vi "TestRFGVRoom.vi"() -> (0 "error out":errorcluster, 2 "Pass":bool)   [LabVIEW 2015]
uses:
  LVClasses/Flags/ColorFlags.ctl
  TypeDef/RoomsActionEnum.ctl
  LVClasses/Room/Room.lvclass/Room.ctl
  LVClasses/Room/Read Flags.lvclass.vi
  LVClasses/Flags/Flags.lvclass
  LVClasses/Room/Room.lvclass
panel:
  out "Read Room JSON 2":string
  out "Read Room JSON 1":string
  out "Read Room 2":T1={"Flag State"=[1, 3, 5, 7]}
  out "Read Flag":string
  out "Write Flag":string
  in  "State":bool[](array[boolean])=[FALSE, FALSE, FALSE, FALSE]
  out "Flags Read 1":T1={"Flag State"=[1, 3, 5, 7]}
  out "Flags Write":T1={"Flag State"=[1, 3, 5, 7]}
  out "Flags Read 2":T1={"Flag State"=[1, 3, 5, 7]}
  in  "FGV Room":i32=102
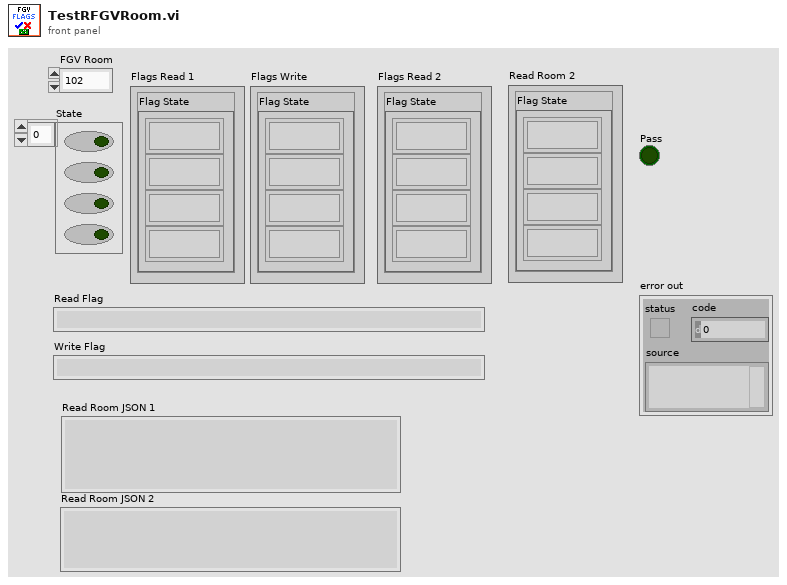
[diagram p1: front panel]
types:
  T1 = typedef "Flags.lvclass/ColorFlags.ctl" = cluster{"Flag State":u8[]}
  T2 = typedef "RoomsActionEnum.ctl" = enum16{"Init", "Add Room", "Remove Room", "Read Room", "Read Flag", "Read Flag State", "Write Flag State", "Read Flag Color", "Write Flag Color", "Read Bed Vacant", "Write Bed Vacant", "Read Personnel", "Add Personnel", "Remove Personnel", "Read Requests", "Add Request", "Remove Request", "Read Beacon ID", "Write Beacon ID", "Write Bed URL", "Read Bed URL", "Read Rooms Numbers", "Write Flag"}
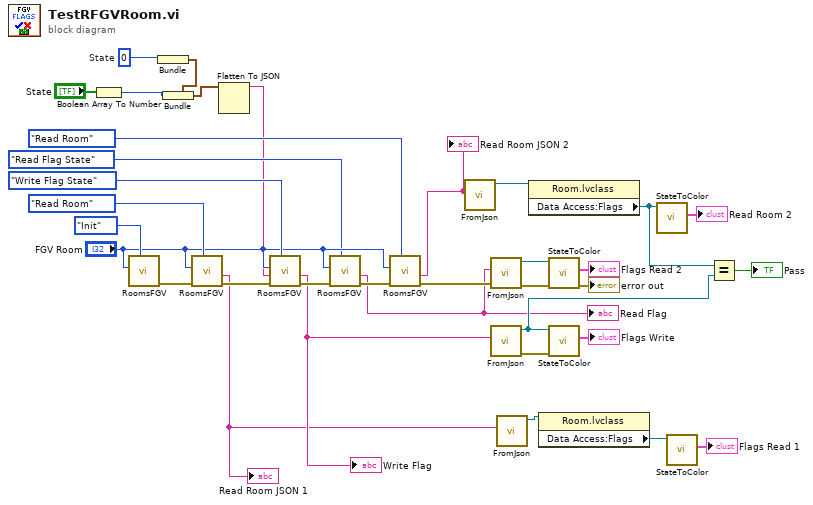
[diagram p0: block diagram]
diagram:
  w5 = u32 0  # State
  n1 = Boolean Array To Number(Boolean array="State") -> (number=w4:u32)
  n2 = call "RoomsFGV.vi"("Actions"=RoomsActionEnum."Init", "Room"="FGV Room") -> ("error out"=w34:errorcluster)  [unwired: 8 in, 1 out]
  n3 = Bundle("State"=w5) -> (w2:cluster{"State":u32})  [unwired: 1 in]
  n4 = Bundle(cluster=w2, "State"=w4) -> (w3:cluster{"State":u32})
  n5 = call "RoomsFGV.vi"("Actions"=RoomsActionEnum."Read Room", "error in (no error)"=w34, "Room"="FGV Room") -> ("error out"=w33:errorcluster, "Data Out"=w12:string)  [unwired: 7 in]
  "Read Room JSON 1" <- w12
  n6 = Flatten To JSON(anything=w3) -> (JSON string=w1:string)  [unwired: 2 in, 1 out]
  n7 = call "RoomsFGV.vi"("Actions"=RoomsActionEnum."Write Flag State", "error in (no error)"=w33, "Data In"=w1, "Room"="FGV Room") -> ("error out"=w32:errorcluster, "Data Out"=w23:string)  [unwired: 6 in]
  "Write Flag" <- w23
  n8 = call "RoomsFGV.vi"("Actions"=RoomsActionEnum."Read Flag State", "error in (no error)"=w32, "Room"="FGV Room") -> ("error out"=w17:errorcluster, "Data Out"=w7:string)  [unwired: 7 in]
  "Read Flag" <- w7
  n9 = call "RoomsFGV.vi"("Actions"=RoomsActionEnum."Read Room", "error in (no error)"=w17, "Room"="FGV Room") -> ("error out"=w29:errorcluster, "Data Out"=w13:string)  [unwired: 7 in]
  "Read Room JSON 2" <- w13
  n10 = call "FromJson.vi"("String"=w13) -> ("Room out"=w8:refnum<class "Room.lvclass">)  [unwired: 9 in, 1 out]
  n11 = call "FromJson.vi"("error in (no error)"=w29, "String"=w7) -> ("error out"=w28:errorcluster, "Flags out"=w14:refnum<class "Flags.lvclass">)  [unwired: 8 in]
  n12 = call "FromJson.vi"("String"=w23) -> ("error out"=w25:errorcluster, "Flags out"=w22:refnum<class "Flags.lvclass">)  [unwired: 9 in]
  n13 = call "FromJson.vi"("String"=w12) -> ("Room out"=w11:refnum<class "Room.lvclass">)  [unwired: 9 in, 1 out]
  n14 = property class="Room.lvclass"(reference=w8) -> ("Data Access:Flags"=w6:refnum<class "Flags.lvclass">)  [unwired: 1 in, 2 out]
  n15 = property class="Room.lvclass"(reference=w11) -> ("Data Access:Flags"=w10:refnum<class "Flags.lvclass">)  [unwired: 1 in, 2 out]
  n16 = call "StateToColor.vi"("error in (no error)"=w28, "Flags in"=w14) -> ("error out"=→"error out":errorcluster, "RoomNumFlags"=→"Flags Read 2":T1)  [unwired: 7 in, 1 out]
  n17 = call "StateToColor.vi"("error in (no error)"=w25, "Flags in"=w22) -> ("RoomNumFlags"=→"Flags Write":T1)  [unwired: 7 in, 2 out]
  n18 = call "StateToColor.vi"("Flags in"=w6) -> ("RoomNumFlags"=→"Read Room 2":T1)  [unwired: 8 in, 2 out]
  n19 = call "StateToColor.vi"("Flags in"=w10) -> ("RoomNumFlags"=→"Flags Read 1":T1)  [unwired: 8 in, 2 out]
  n20 = Equal?(x=w6, y=w22) -> (x = y?=→"Pass":bool)
